vi "JudgeYear.vi"(10 "DataMonth":i32) -> (2 "DataYear":i32)   [LabVIEW 2012]
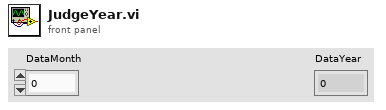
[diagram p1: front panel]
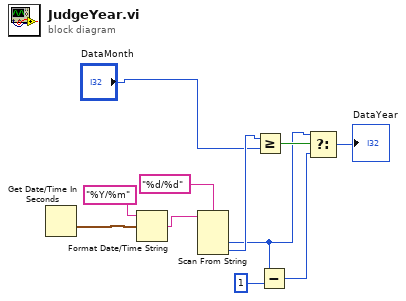
[diagram p0: block diagram]
diagram:
  n1 = Get Date/Time In Seconds() -> (seconds since 1Jan1904=w1:timestamp)
  n2 = Format Date/Time String(time format string (%c)="%Y/%m", seconds (now)=w1) -> (date/time string=w10:string)  [unwired: 1 in]
  n3 = Scan From String(format string="%d/%d", input string=w10) -> (output 1=w5:i32, output 2=w8:i32)  [unwired: 4 in, 3 out]
  n4 = Greater Or Equal?(x=w8, y="DataMonth") -> (x >= y?=w6:bool)
  n5 = Subtract(x=w5, y=1) -> (x-y=w3:i32)
  n6 = Select(t=w5, s=w6, f=w3) -> (s? t:f=→"DataYear":i32)
